vi "Get Output.vi"(11 "AER in":refnum<class "AER.lvclass">) -> (1 "AvePC":dbl, 2 "PCs":dbl[](array[numeric]), 3 "AER out":refnum<class "AER.lvclass">)   [LabVIEW 2013, in "AER.lvclass"]
uses:
  AER.lvclass
  Controls/Type of Neuron.ctl
  AER.lvclass/AER.ctl
panel:
  out "No PC":i32
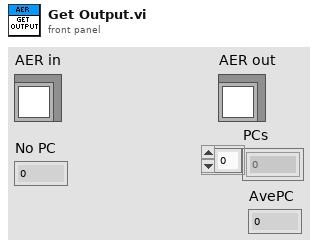
[diagram p1: front panel]
types:
  T1 = typedef "Type of Neuron.ctl" = enum16{"MF", "BA", "GO", "GC", "PC", "LU", "Glia (Dummy)"}
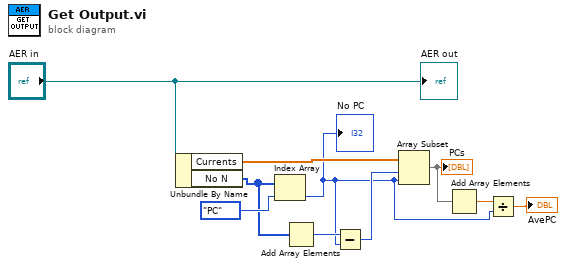
[diagram p0: block diagram]
diagram:
  n1 = Unbundle By Name("AER in") -> ("Currents"=w9:dbl[], "No N"=w7:i32[])
  n2 = Index Array(array=w7, index=Type_of_Neuron."PC" ("Type of Neuron")) -> (element=w1:i32)
  "No PC" <- w1
  n3 = Add Array Elements(numeric array=w7) -> (sum=w6:i32)
  n4 = Subtract(x=w6, y=w1) -> (x-y=w5:i32)
  n5 = Array Subset(array=w9, index=w5, length=w1) -> (w4:dbl[])
  "PCs" <- w4
  n6 = Add Array Elements(numeric array=w4) -> (sum=w3:dbl)
  n7 = Divide(x=w3, y=w1) -> (x/y=→"AvePC":dbl)
  "AER out" <- "AER in"
